vi "Get PinNames List.vi"(11 "error in (no error)":errorcluster) -> (4 "PinNames Label":string[](array[string]), 15 "error out":errorcluster)   [LabVIEW 2021, in "Converter Reusables.lvlib"]
uses:
  Converter Reusables.lvlib
  controls/Dictionary States.ctl
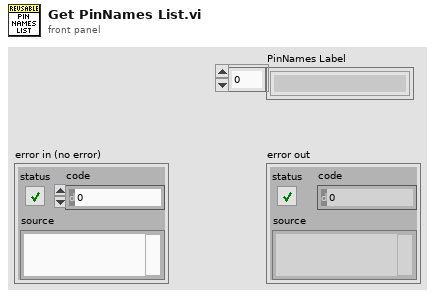
[diagram p1: front panel]
types:
  T1 = typedef "Converter Reusables.lvlib/Dictionary States.ctl" = enum16{"Set", "Get", "Delete", "Delete All"}
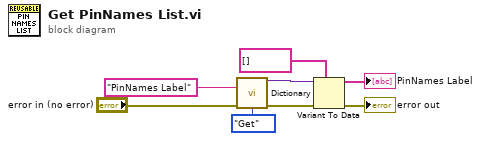
[diagram p0: block diagram]
diagram:
  n1 = call "Dictionary.vi"("Key"="PinNames Label", "error in (no error)"="error in (no error)", "Dict States"=Dictionary_States."Get") -> ("Variant_Out"=w3:variant, "error out"=w4:errorcluster)  [unwired: 11 in]
  n2 = Variant To Data(error in=w4, type=string[] [], Variant=w3) -> (data=→"PinNames Label":string[], error out=→"error out":errorcluster)
